vi "8-2.vi"() -> ()   [LabVIEW 2022 SP3, in "AoC22.lvlib"]
uses:
  AoC22.lvlib
  Tree.ctl
  <vilib>/IlluminatedG/lv-stream/Stream.lvlib
panel:
  out "x = y?":bool
  out "max index(es)":i32[](array[numeric])
  out "max value":i32
  out "Score":i32[][](array[numeric])
  out "Array":T1[][](array[typedef])
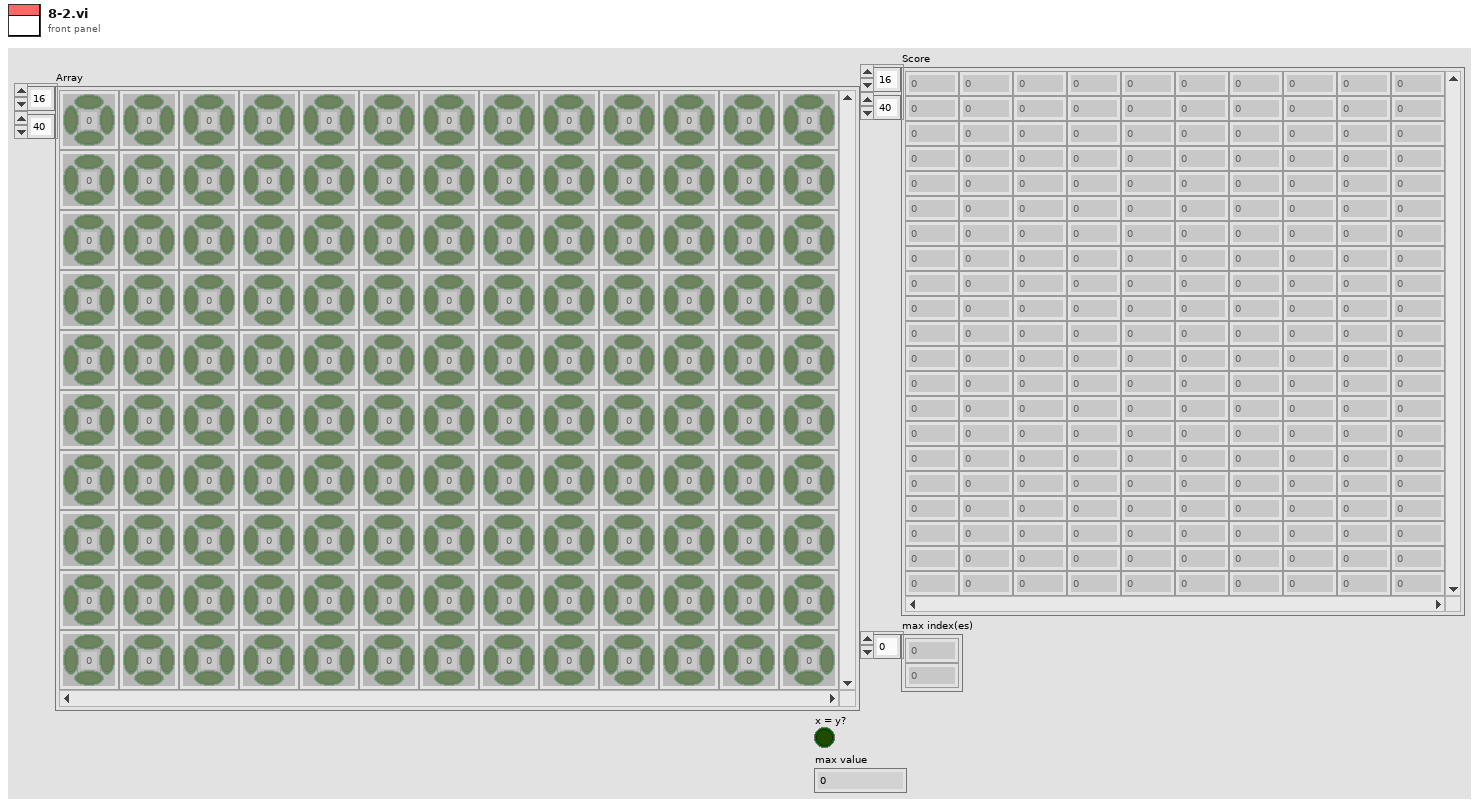
[diagram p1: front panel]
types:
  T1 = typedef "AoC22.lvlib/Tree.ctl" = cluster{"Height":i32, "Up":bool, "Left":bool, "Down":bool, "Right":bool}
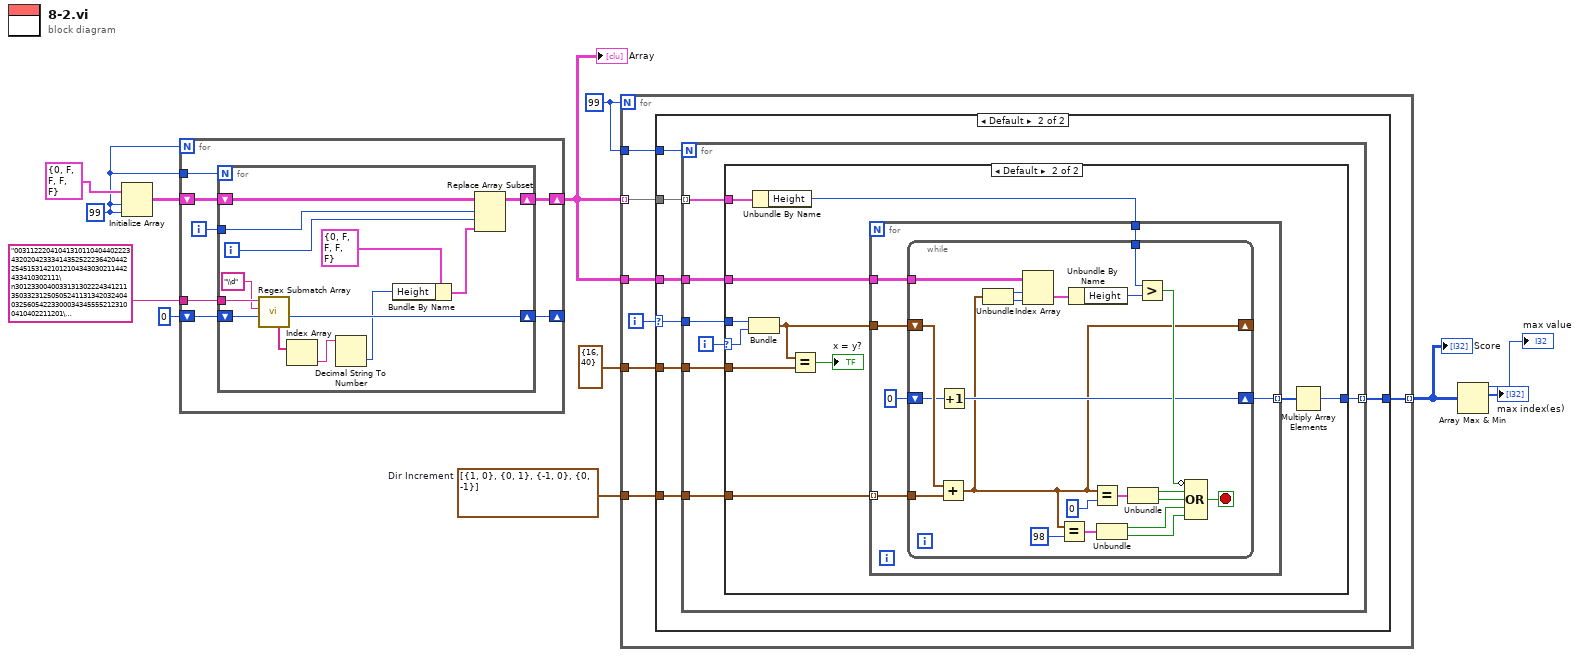
[diagram p0: block diagram]
diagram:
  w6 = cluster{i32, i32}[] [{1, 0}, {0, 1}, {-1, 0}, {0, -1}]  # Dir Increment
  w7 = 99
  w10 = 99 ("dimension size")
  n1 = Initialize Array(T1 {"Height"=0, "Up"=FALSE, "Left"=FALSE, "Down"=FALSE, "Right"=FALSE} ("Tree"), w10, w10) -> (w11:T1[][])
  n2 = for {
    N: w10 -> [_]
    shift-right: [w16] -> w1
    shift-left: w11 -> [w19]
    tunnel: w10 -> [w18]
    tunnel: "003112220410413101104044022234320204233341435252223642044225451531421012104343030211442433410302111\n301233004003313130222434121135033231250505241131342032404032560542233000343455552123100410402211201\n111301041221333142533352050250154136146324550411565615444115604102531135302000320033233340431313123\n011312210420442043155233305201305643445224334303310253225205601265233454400214114322131420224022313\n130102441231200141254202121022423405224443210463250415204410624313613034320040015223211432442333110\n133121132322223054104323242043651144066341346000104210124535555236324451132555525220523220023202433\n..." -> [w15]
    shift-right: [w14] -> _
    shift-left: 0 ("offset past match") -> [w13]
    i -> [w17]
    n3 = for {
      N: w18 -> [_]
      shift-right: [w31] -> w16
      shift-left: w19 -> [w32]
      tunnel: w17 -> [w29]
      tunnel: w15 -> [w28]
      shift-right: [w26] -> w14
      shift-left: w13 -> [w25]
      i -> [w30]
      n4 = call <vilib>:"Regex Submatch Array.vi"("offset (0)"=w25, "regular expression"="\\d", "string"=w28) -> ("offset past match"=w26:i32, "matches"=w24:string[])  [unwired: 6 in, 1 out]
      n5 = Index Array(array=w24) -> (element=w23:string)  [unwired: 1 in]
      n6 = Decimal String To Number(string=w23) -> (number=w20:i32)  [unwired: 2 in, 1 out]
      n7 = Bundle By Name(cluster=T1 {"Height"=0, "Up"=FALSE, "Left"=FALSE, "Down"=FALSE, "Right"=FALSE} ("new element/subarray"), "Height"=w20) -> (w21:T1)
      n8 = Replace Array Subset(array=w32, new element=w21, index (row)=w29, index (col)=w30) -> (w31:T1[][])
    }
  }
  "Array" <- w1
  n9 = for {
    N: w7 -> [_]
    tunnel: w1 -> [w39] mode=indexing
    tunnel: w7 -> [w37]
    tunnel: [w36] -> w5 mode=indexing
    tunnel: w6 -> [w35]
    tunnel: w1 -> [w34]
    tunnel: cluster{i32, i32} {16, 40} -> [w33]
    i -> [w38]
    n10 = case shown="Default" w38 {
      selector: w38 -> [_ w45]
      tunnel: w39 -> [_ w46]
      tunnel: w37 -> [_ w44]
      tunnel: [_ w43] -> w36
      tunnel: w35 -> [_ w42]
      tunnel: w34 -> [_ w41]
      tunnel: w33 -> [_ w40]
      frame 0, 98 {
      }
      frame Default {
        n11 = for {
          N: w44 -> [_]
          tunnel: w46 -> [w51] mode=indexing
          tunnel: w45 -> [w52]
          tunnel: [w50] -> w43 mode=indexing
          tunnel: w42 -> [w49]
          tunnel: w41 -> [w48]
          tunnel: w40 -> [w47]
          i -> [w53]
          n12 = case shown="Default" w53 {
            selector: w53 -> [_ w63]
            tunnel: w52 -> [_ w64]
            tunnel: w51 -> [_ w62]
            tunnel: [_ w58] -> w50
            tunnel: w49 -> [_ w60]
            tunnel: w48 -> [_ w61]
            tunnel: w47 -> [_ w55]
            frame 0, 98 {
            }
            frame Default {
              n13 = Bundle(w64, w63) -> (w56:cluster{i32, i32})  [unwired: 1 in]
              n14 = Unbundle By Name(w62) -> ("Height"=w57:i32)
              n15 = Equal?(x=w56, y=w55) -> (x = y?=→"x = y?":bool)
              n16 = for {
                tunnel: w61 -> [w66]
                tunnel: w60 -> [w69] mode=indexing
                tunnel: w56 -> [w67]
                tunnel: [w68] -> w59 mode=indexing
                tunnel: w57 -> [w65]
                n17 = while {
                  shift-right: [w72] -> w68
                  shift-left: 0 -> [w73]
                  tunnel: w69 -> [w91]
                  shift-right: [w71] -> _
                  shift-left: w67 -> [w80]
                  tunnel: w66 -> [w81]
                  tunnel: w65 -> [w75]
                  stop <- w82 stop-if-true
                  n18 = Add(x=w80, y=w91) -> (x+y=w71:cluster{i32, i32})
                  n19 = Increment(x=w73) -> (x+1=w72:i32)
                  n20 = Unbundle(w71) -> (w79:i32, w78:i32)
                  n21 = Index Array(array=w81, index (row)=w79, index (col)=w78) -> (element=w77:T1)
                  n22 = Equal?(x=w71, y=98) -> (x = y?=w88:cluster{bool, bool})
                  n23 = Unbundle By Name(w77) -> ("Height"=w76:i32)
                  n24 = Equal?(x=w71, y=0) -> (x = y?=w87:cluster{bool, bool})
                  n25 = Unbundle(w88) -> (w84:bool, w83:bool)
                  n26 = Unbundle(w87) -> (w86:bool, w85:bool)
                  n27 = Greater?(x=w75, y=w76) -> (0:w74:bool)
                  n28 = Compound Arithmetic op=OR(invert w74, w86, w85, w84, w83) -> (w82:bool)
                }
              }
              n29 = Multiply Array Elements(1:w59) -> (0:w58:i32)
            }
          }
        }
      }
    }
  }
  "Score" <- w5
  n30 = Array Max & Min(array=w5) -> (max value=→"max value":i32, max index (indices)=→"max index(es)":i32[])  [unwired: 2 out]
